vi "Create Test Pattern.vi"() -> ()   [LabVIEW 2016]
uses:
  SoftwareLockin/Lockin Parameters.ctl
  <vilib>/Analysis/NI_AALBase.lvlib
panel:
  in  "channel name(s) in (Untitled)":string
  in  "Harmonics":i32[](array[numeric])=[1, 2, 3]
  in  "Sample rate":dbl=9000000.0
  in  "Samples":i32=10000
  in  "Lockin parameters":T1={"Frequency"=100000.0, "Phase"=0.0, "Syncronous"=TRUE, "Points per sine wave"=90, "DDS"=FALSE, "Frequency word"=0, "Phase word"=0, "DDS modulus"=15120, "DDS clock"=125000000.0} {"DDS clock" format="%_17pHz"; "DDS modulus" format="0x%x (%d)"; "Phase" format="%#_gdeg"; "Frequency" format="%_17pHz"}
  out "Waveform Graph":dbl[](graph)
  in  "File Path Control":path=path "C:/Data/test.tdms"
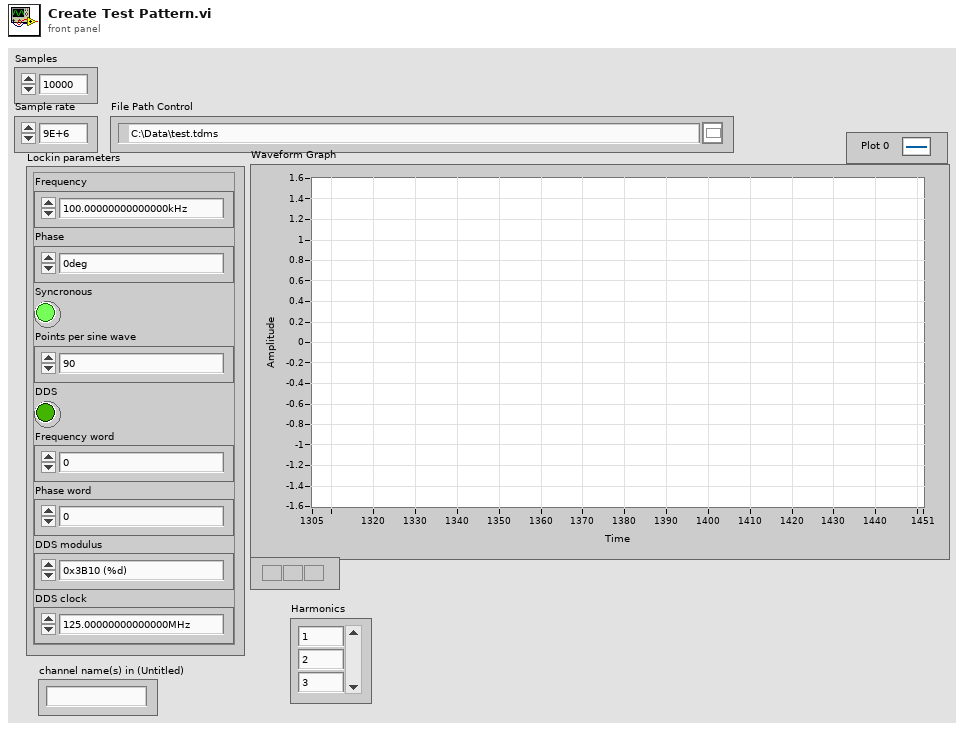
[diagram p1: front panel]
types:
  T1 = typedef "Lockin Parameters.ctl" = cluster{"Frequency":dbl, "Phase":dbl, "Syncronous":bool, "Points per sine wave":i32, "DDS":bool, "Frequency word":u32, "Phase word":u32, "DDS modulus":i64, "DDS clock":dbl}
  T2 = enum16{"open", "open or create", "create or replace", "create", "open (read-only)"}
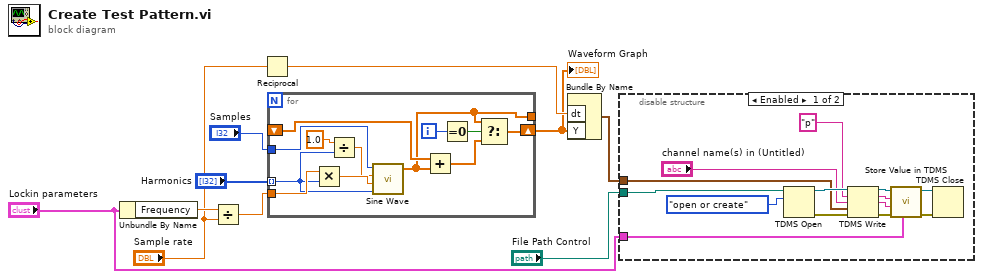
[diagram p0: block diagram]
diagram:
  n1 = Unbundle By Name("Lockin parameters") -> ("Frequency"=w7:dbl)
  n2 = Divide(x=w7, y="Sample rate") -> (x/y=w8:dbl)
  n3 = Reciprocal(x="Sample rate") -> (1/x=w5:dbl)
  n4 = for {
    tunnel: "Samples" -> [w22]
    tunnel: w8 -> [w20]
    tunnel: [w15] -> _
    tunnel: "Harmonics" -> [w11] mode=indexing
    shift-right: [w13] -> w3
    shift-left: _ -> [w18]
    i -> [w17]
    n5 = Multiply(x=w20, y=w11) -> (x*y=w19:dbl)
    n6 = Divide(x=1.0 ("amplitude"), y=w11) -> (x/y=w12:dbl)
    n7 = call <vilib>:"Sine Wave.vi"("samples"=w22, "amplitude"=w12, "frequency"=w19, "phase in"=w11) -> ("sine wave"=w15:dbl[])  [unwired: 1 in, 2 out]
    n8 = Add(x=w18, y=w15) -> (x+y=w14:dbl[])
    n9 = Equal To 0?(x=w17) -> (x = 0?=w16:bool)
    n10 = Select(t=w15, s=w16, f=w14) -> (s? t:f=w13:dbl[])
  }
  "Waveform Graph" <- w3
  n11 = Bundle By Name("dt"=w5, "Y"=w3) -> (w2:waveform(dbl))  [unwired: 1 in]
  n12 = disable-structure shown="Enabled" {
    disable-tunnel: "File Path Control" -> [w36 _]
    disable-tunnel: w2 -> [w32 _]
    disable-tunnel: "Lockin parameters" -> [w25 _]
    frame Enabled {
      n13 = TDMS Open(10:T2."open or create" ("operation (0:open)"), 11:w36) -> (0:w29:errorcluster, 3:w34:refnum<k34>)  [unwired: 5 in]
      n14 = TDMS Write(0:w34, 5:"p" ("group name in (Untitled)"), 7:"channel name(s) in (Untitled)", 9:w32, 11:w29) -> (4:w30:refnum<k34>, 6:w27:string, 8:w26:string, 15:w28:errorcluster)  [unwired: 1 in]
      n15 = call "Store Value in TDMS.vi"("Value"=w25, "Error In"=w28, "channel name"=w26, "group name"=w27, "tdms file"=w30) -> ("Error Out"=w23:errorcluster, "tdms file out"=w24:refnum<k34>)  [unwired: 3 in, 2 out]
      n16 = TDMS Close(8:w23, 11:w24) -> ()  [unwired: 2 out]
    }
    frame Disabled {
    }
  }
